vi "Panel.vi"(11 "BooleanIndicatorEditorPanel in":refnum<class "BooleanIndicatorEditorPanel.lvclass">) -> ()   [LabVIEW 2020, in "VolatusGUIControls.lvlib" / "BooleanIndicatorEditorPanel.lvclass"]
uses:
  BooleanIndicatorEditorPanel.lvclass
  BooleanIndicatorEditorPanel.lvclass/BooleanIndicatorEditorPanel.ctl
  lv-oopanel/OOPanel/Panel/Basic UI State.ctl
  lv-oopanel/OOPanel/Panel/Panel.lvclass
  lv-oopanel/OOPanel/OOPanel.lvlib
  VolatusGUIEditorCore/ElementEditorPanel/ElementEditorPanel.lvclass
  lv-autocomplete/AutoComplete/AutoComplete/AutoComplete.lvclass
  VolatusGUIEditorCore/VolatusGUIEditorCore.lvlib
  C:/dev/lv20CE/relink/volatus-gui-controls/VolatusGUIEditorCore/ElementEditorPanel/ElementEditorPanel.lvclass
  C:/dev/lv20CE/relink/lv-oopanel/OOPanel/Panel/Panel.lvclass
  C:/dev/lv20CE/relink/volatus-gui-controls/VolatusGUIControls/BooleanIndicatorEditorPanel/BooleanIndicatorEditorPanel.lvclass
panel:
  in  "Text":bool
  in  "Top":i32
  in  "Left":i32
  in  "Height":u16
  in  "Width":u16
  in  "Label Text Color":u32(colorbox) caption="Color"
  in  "Text Color":u32(colorbox) caption="Color"
  in  "Label Visible":bool caption="Visible"
  in  "Label":string
  in  "Multi":bool
  in  "Channel":string
  in  "True Color":u32(colorbox)
  in  "False Color":u32(colorbox)
  in  "True Text":string
  in  "False Text":string
  # "Label"
  # "False"
  # "True"
  # "LED"
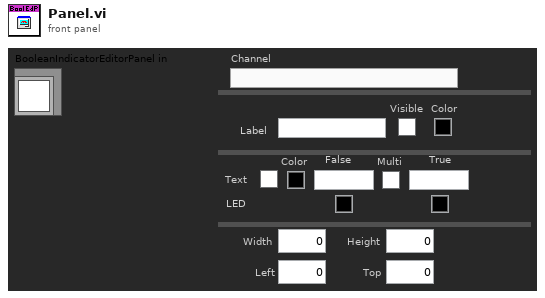
[diagram p1: front panel]
types:
  T1 = typedef "OOPanel.lvlib/Panel.lvclass/Basic UI State.ctl" = enum16{"Init", "Run", "Close"}
  T2 = typedef "VolatusGUIEditorCore.lvlib/ElementEditorPanel.lvclass/Incoming Events.ctl" = cluster{"Update Control":refnum<user-event>}
  T3 = typedef "OOPanel.lvlib/Panel.lvclass/Panel Events.ctl" = cluster{"Visbility":refnum<user-event>, "Close":refnum<user-event>}
  T4 = typedef "VolatusGUIControls.lvlib/BooleanIndicatorEditorPanel.lvclass/Props.ctl" = cluster{"JSON":T5, "Label":T6, "Position":T7, "Width":u16, "Height":u16, "Boolean Colors":T8, "Boolean Text Props":T9}
  T5 = typedef "VolatusGUIControls.lvlib/BooleanIndicatorEditorPanel.lvclass/JSON Props.ctl" = cluster{"Channel":string}
  T6 = typedef "VolatusGUIEditorCore.lvlib/Label Props.ctl" = cluster{"Text":string, "Text Color":u32, "Visible":bool}
  T7 = typedef "VolatusGUIEditorCore.lvlib/Position Props.ctl" = cluster{"Left":i32, "Top":i32}
  T8 = typedef "VolatusGUIEditorCore.lvlib/Boolean Color Props.ctl" = cluster{"False":u32, "True":u32}
  T9 = typedef "VolatusGUIEditorCore.lvlib/Boolean Text Props.ctl" = cluster{"Color":u32, "MultiString":bool, "False":string, "True":string, "Visible":bool}
  T10 = typedef "OOPanel.lvlib/Visibility State.ctl" = enum16{"Idle", "Closed", "Hidden", "Visible", "Subpanel", "Hidden Subpanel"}
  T11 = cluster{"Text Color":u32, "Multi":bool, "False Text":string, "True Text":string, "Text":bool}
  T12 = cluster{"Label":string, "Label Text Color":u32, "Label Visible":bool}
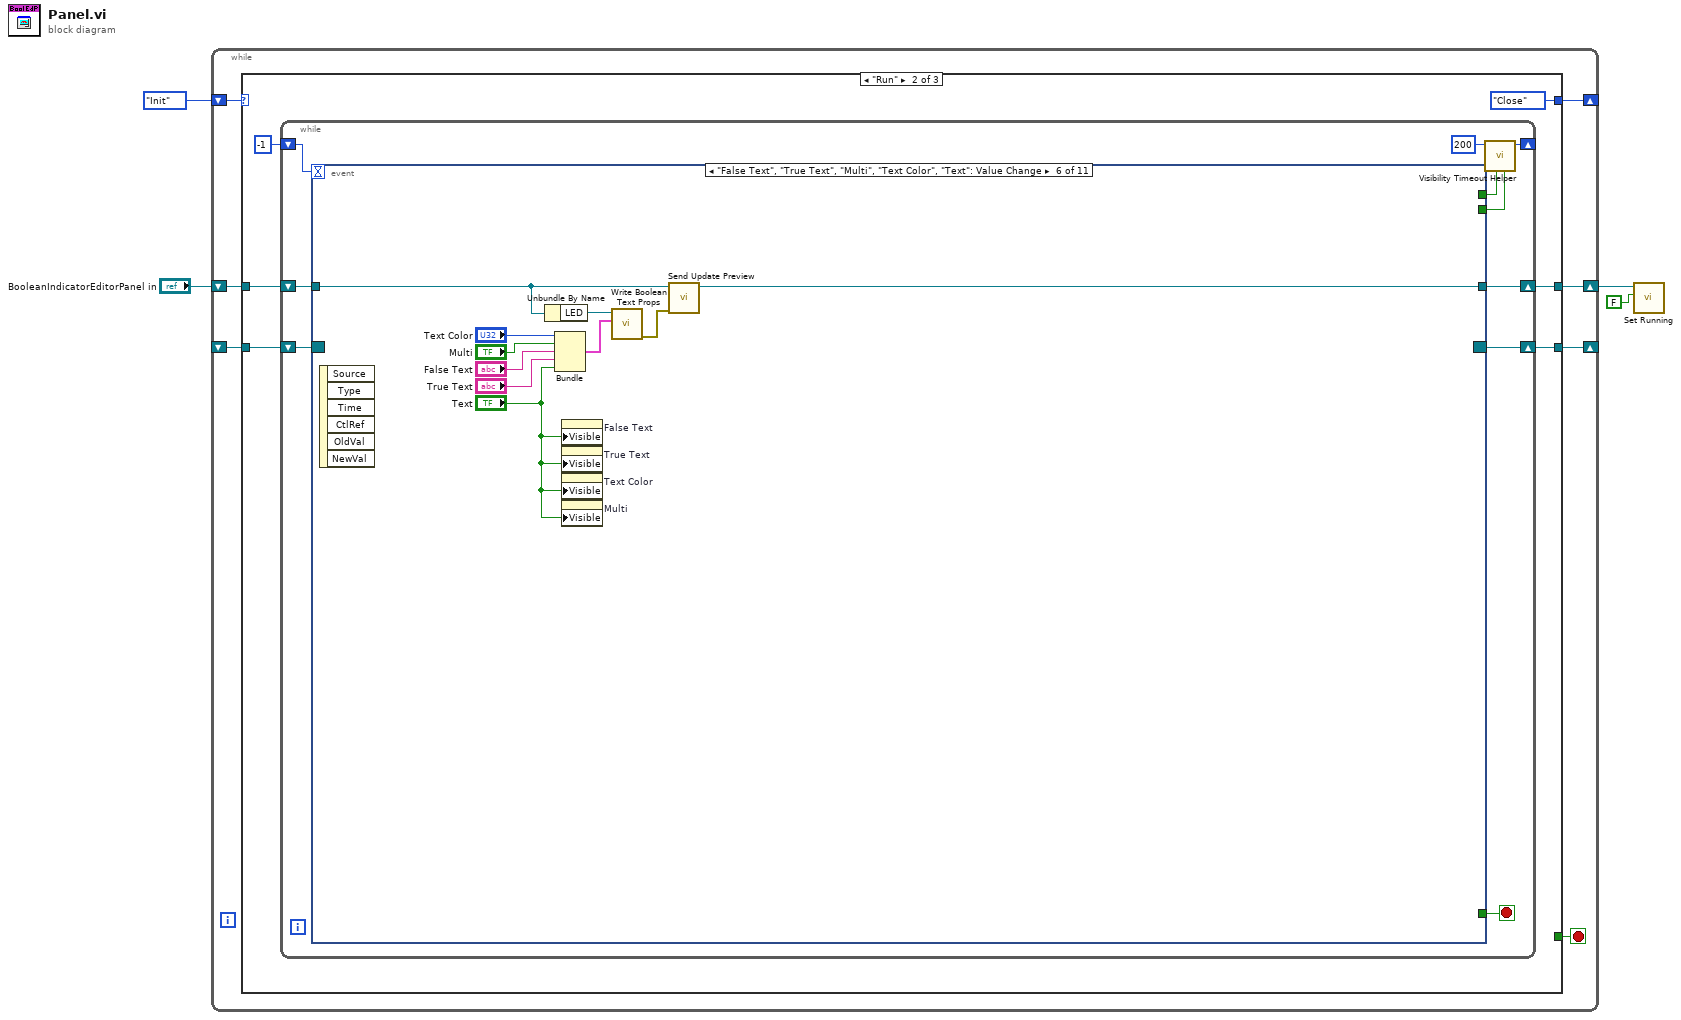
[diagram p0: block diagram]
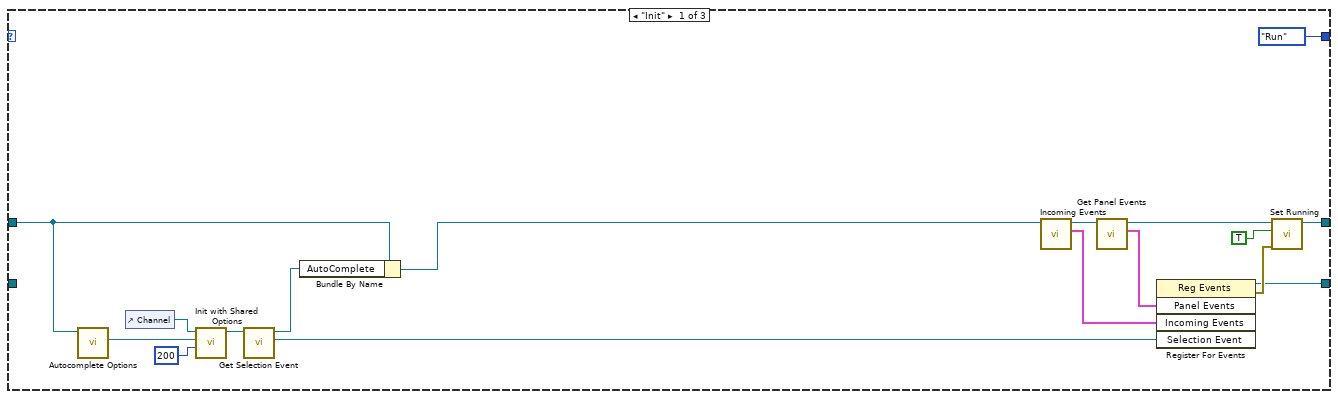
[diagram p2: hidden frame]
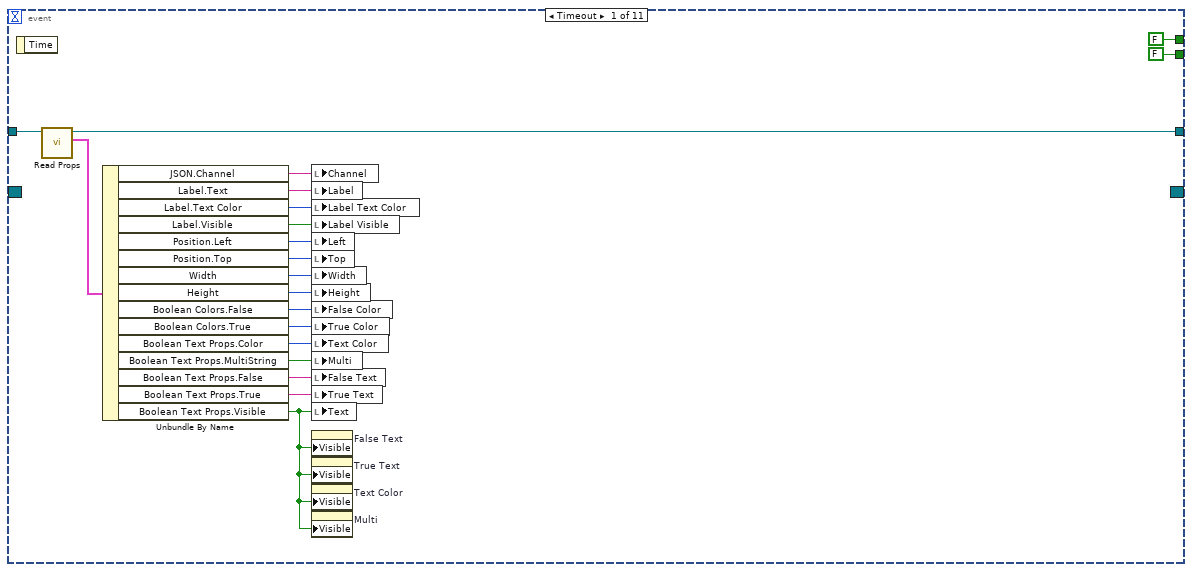
[diagram p3: hidden frame]
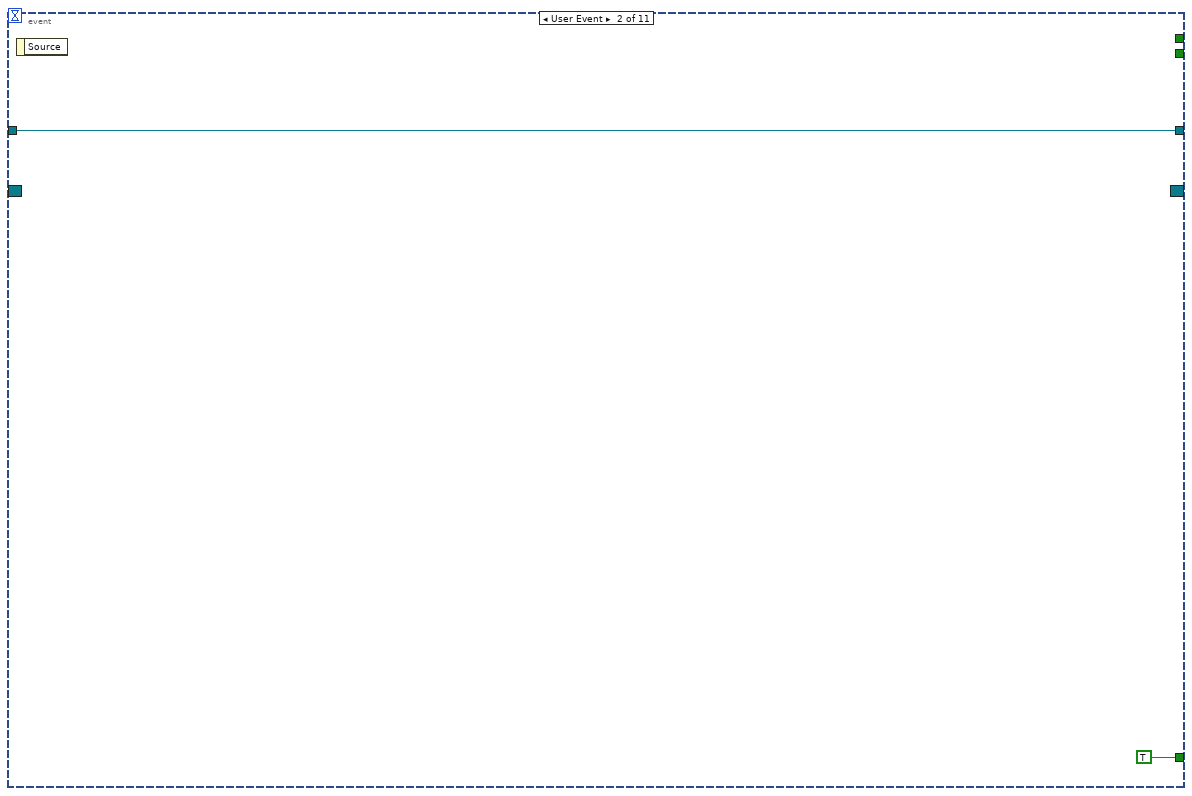
[diagram p4: hidden frame]
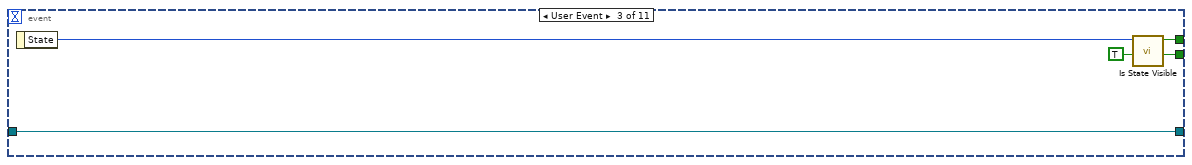
[diagram p5: hidden frame]
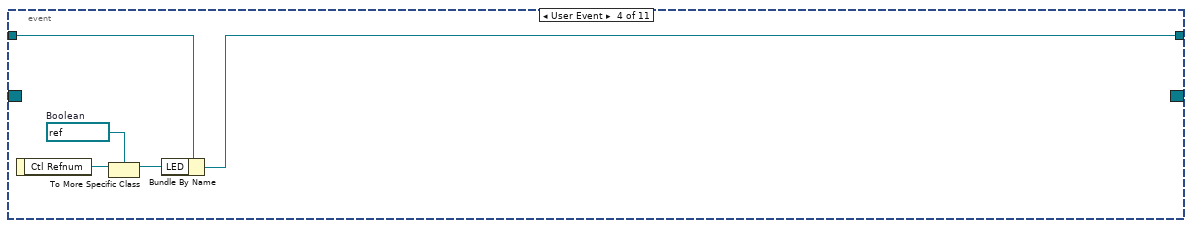
[diagram p6: hidden frame]
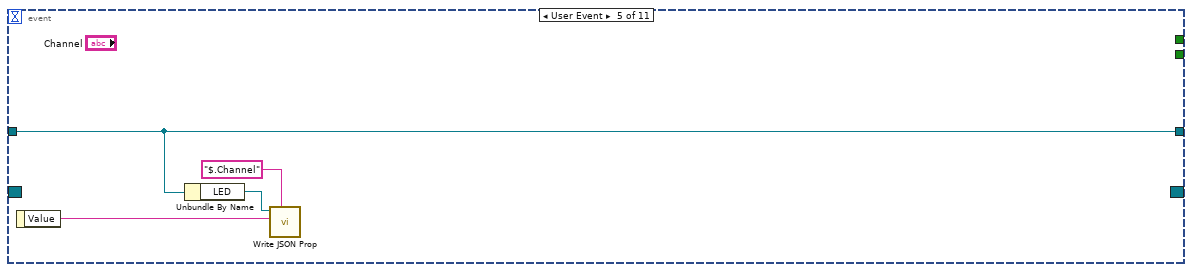
[diagram p7: hidden frame]
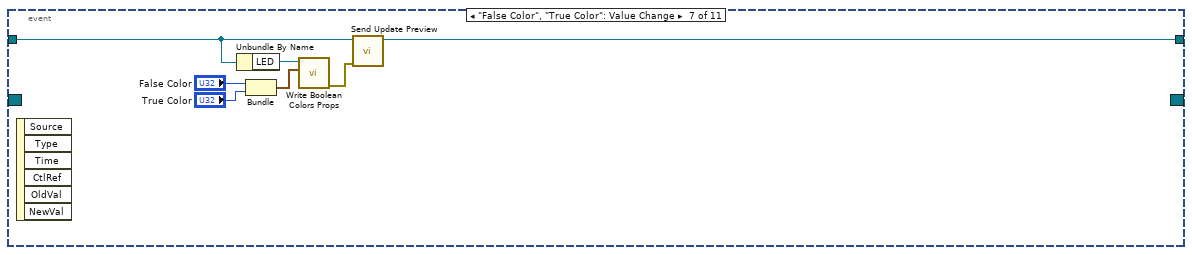
[diagram p8: hidden frame]
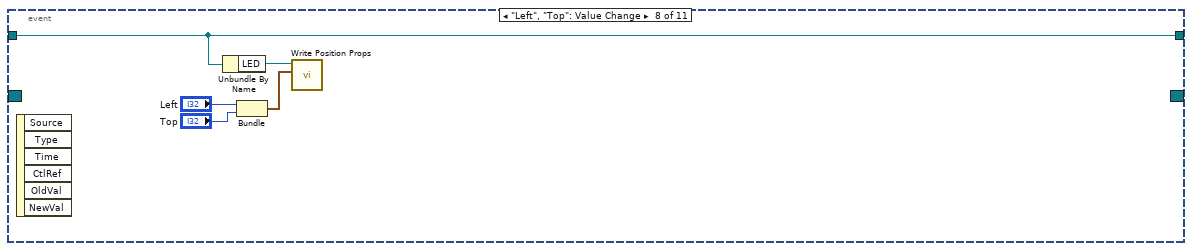
[diagram p9: hidden frame]
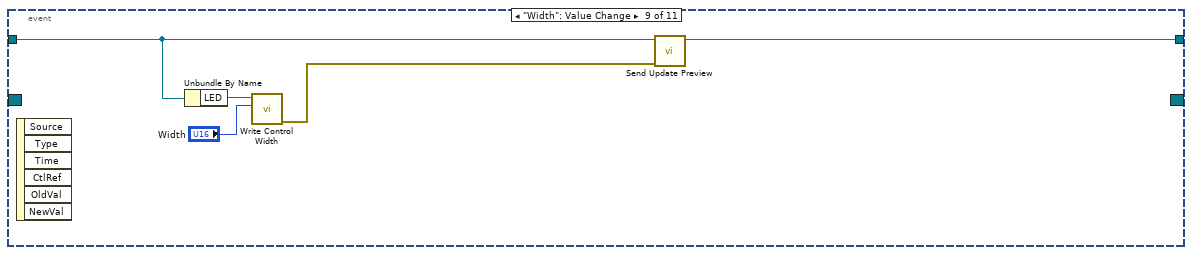
[diagram p10: hidden frame]
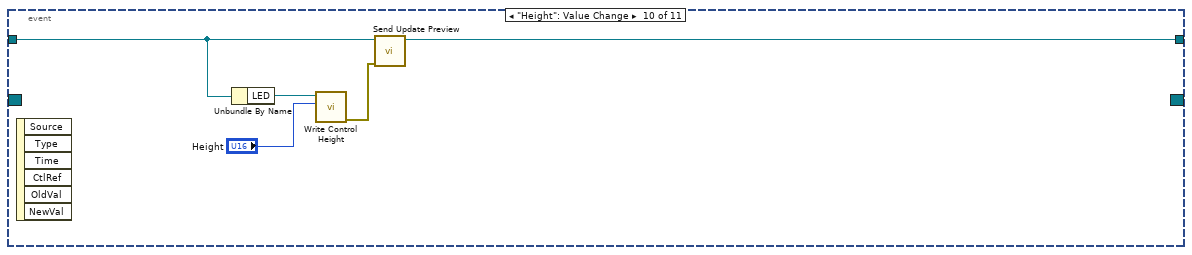
[diagram p11: hidden frame]
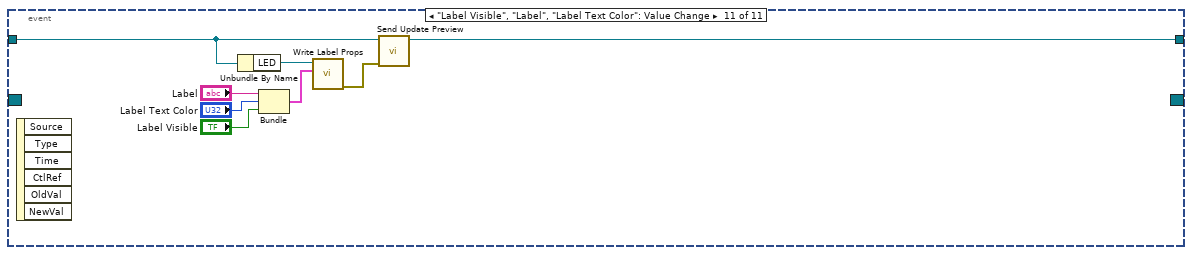
[diagram p12: hidden frame]
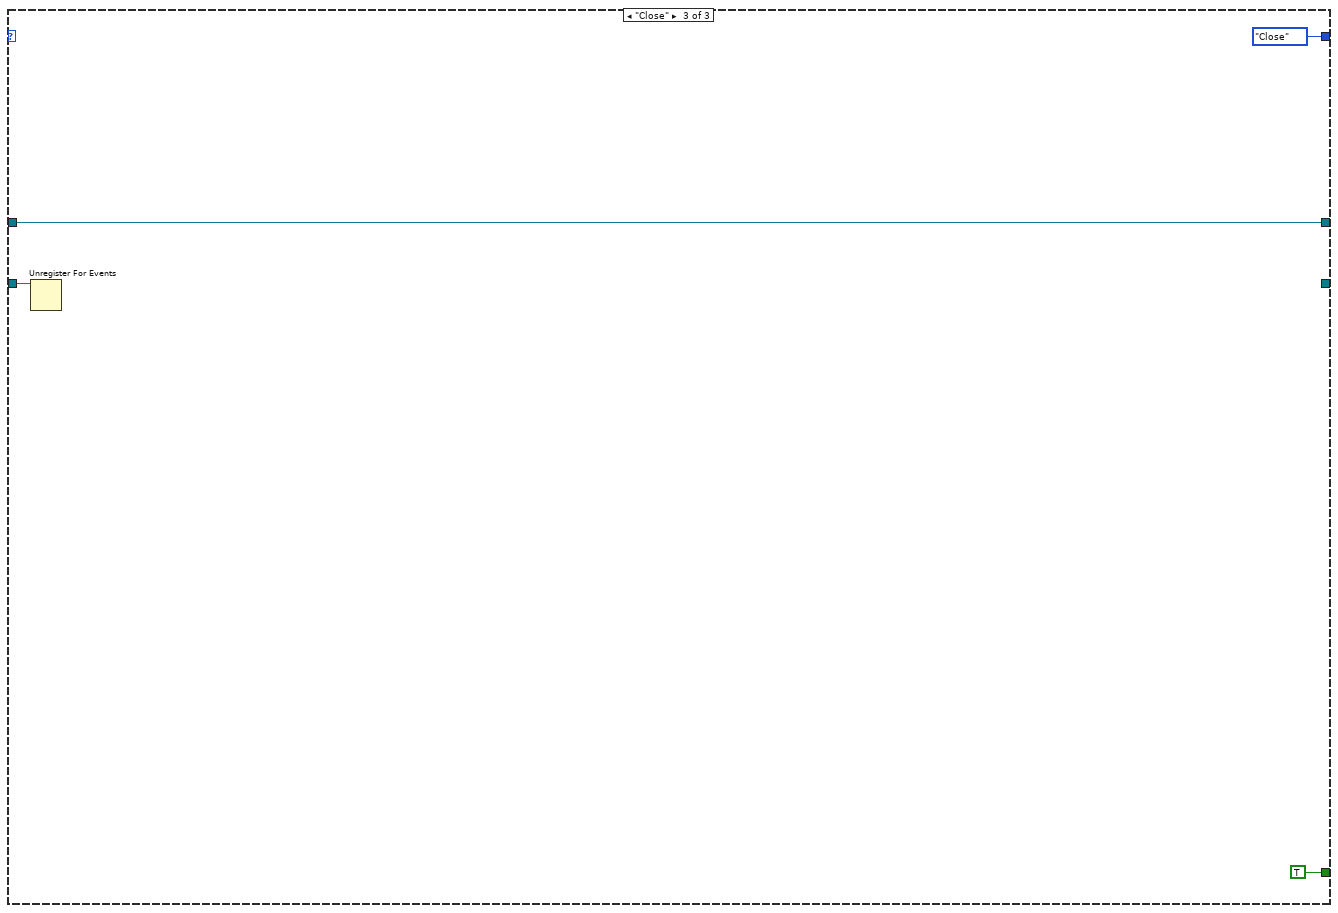
[diagram p13: hidden frame]
diagram:
  n1 = while {
    shift-right: [w10] -> _
    shift-left: _ -> [w11]
    shift-right: [w8] -> _
    shift-left: Basic_UI_State."Init" ("Basic UI State") -> [w9]
    shift-right: [w6] -> w4
    shift-left: "BooleanIndicatorEditorPanel in" -> [w5]
    stop <- w7 stop-if-true
    n2 = case shown="\"Run\"" w9 {
      tunnel: w11 -> [_ w34 w121]
      tunnel: [w25 w32 _] -> w10
      tunnel: [Basic_UI_State."Run" ("Basic UI State") Basic_UI_State."Close" ("Basic UI State") Basic_UI_State."Close" ("Basic UI State")] -> w8
      tunnel: [_ _ TRUE] -> w7
      tunnel: [w24 w29 w120] -> w6
      tunnel: w5 -> [w16 w30 w120]
      frame "Init" {
        n3 = call "Autocomplete Options.vi"("ElementEditorPanel in"=w16) -> ("Autocomplete Options"=w19:refnum<class "Shared Options.lvclass">)  [unwired: 10 in]
        n4 = control-ref of="Channel"() -> (w15:refnum<vi>)
        n5 = call "Init with Shared Options.vi"("Height (200)"=i16 200, "Shared Options"=w19, "Str Refnum"=w15) -> ("AutoComplete out"=w18:refnum<class "AutoComplete.lvclass">)  [unwired: 7 in, 1 out]
        n6 = call "Get Selection Event.vi"("AutoComplete in"=w18) -> ("Selection Event"=w12:refnum<user-event>, "AutoComplete"=w13:refnum<class "AutoComplete.lvclass">)  [unwired: 9 in]
        n7 = Bundle By Name(cluster=w16, "AutoComplete"=w13) -> (w14:refnum<class "BooleanIndicatorEditorPanel.lvclass">)
        n8 = call "Incoming Events.vi"("ElementEditorPanel in"=w14) -> ("Incoming Events"=w20:T2, "ElementEditorPanel out"=w21:refnum<class "BooleanIndicatorEditorPanel.lvclass">)  [unwired: 9 in]
        n9 = call "Get Panel Events.vi"("Panel in"=w21) -> ("Panel Events"=w22:T3, "Panel out"=w23:refnum<class "BooleanIndicatorEditorPanel.lvclass">)  [unwired: 8 in, 1 out]
        n10 = register-events(w22, w20, w12) -> (reference out=w25:refnum<event-registration>, error out=w27:errorcluster)  [unwired: 2 in]
        n11 = call "Set Running.vi"("error in (no error)"=w27, "Running"=TRUE, "Panel in"=w23) -> ("Panel out"=w24:refnum<class "BooleanIndicatorEditorPanel.lvclass">)  [unwired: 7 in, 1 out]
      }
      frame "Run" {
        n12 = while {
          shift-right: [w40] -> w32
          shift-left: w34 -> [w41]
          shift-right: [w43] -> _
          shift-left: -1 ("Timeout") -> [w42]
          shift-right: [w35] -> w29
          shift-left: w30 -> [w36]
          stop <- w37 stop-if-true
          n13 = event shown="[5] \"False Text\", \"True Text\", \"Multi\", \"Text Color\", \"Text\": Value Change" {
            selector: w41 -> [_ _ _ _ _ _ _ _ _ _ _]
            dyn-events: [_ _ _ _ _ _ _ _ _ _ _] -> w40
            timeout: w42 -> [_ _ _ _ _ _ _ _ _ _ _]
            tunnel: [FALSE _ w69 _ _ _ _ _ _ _ _] -> w39
            tunnel: [FALSE _ TRUE _ _ _ _ _ _ _ _] -> w38
            tunnel: [_ TRUE _ _ _ _ _ _ _ _ _] -> w37
            tunnel: w36 -> [w61 w65 w67 w75 w77 w84 w93 w98 w105 w110 w115]
            tunnel: [w62 w65 w67 w72 w77 w82 w91 w98 w103 w108 w113] -> w35
            event Timeout {
              n14 = event-data() -> ()  [unwired: 1 in, 1 out]
              n15 = call "Read Props.vi"("BooleanIndicatorEditorPanel in"=w61) -> ("Props"=w60:T4, "BooleanIndicatorEditorPanel out"=w62:refnum<class "BooleanIndicatorEditorPanel.lvclass">)  [unwired: 8 in, 1 out]
              n16 = Unbundle By Name(w60) -> ("JSON.Channel"=w59:string, "Label.Text"=w58:string, "Label.Text Color"=w57:u32, "Label.Visible"=w56:bool, "Position.Left"=w55:i32, "Position.Top"=w54:i32, "Width"=w53:u16, "Height"=w52:u16, "Boolean Colors.False"=w51:u32, "Boolean Colors.True"=w50:u32, "Boolean Text Props.Color"=w49:u32, "Boolean Text Props.MultiString"=w48:bool, "Boolean Text Props.False"=w47:string, "Boolean Text Props.True"=w46:string, "Boolean Text Props.Visible"=w45:bool)
              n17 = local write "Channel"(w59) -> ()
              n18 = local write "Label"(w58) -> ()
              n19 = local write "Label Text Color"(w57) -> ()
              n20 = local write "Label Visible"(w56) -> ()
              n21 = local write "Left"(w55) -> ()
              n22 = local write "Top"(w54) -> ()
              n23 = local write "Width"(w53) -> ()
              n24 = local write "Height"(w52) -> ()
              n25 = local write "False Color"(w51) -> ()
              n26 = local write "True Color"(w50) -> ()
              n27 = local write "Text Color"(w49) -> ()
              n28 = local write "Multi"(w48) -> ()
              n29 = local write "False Text"(w47) -> ()
              n30 = local write "True Text"(w46) -> ()
              n31 = local write "Text"(w45) -> ()
              n32 = property on="False Text" class="Str"("Visible"=w45) -> ()  [unwired: 2 in, 2 out]
              n33 = property on="True Text" class="Str"("Visible"=w45) -> ()  [unwired: 2 in, 2 out]
              n34 = property on="Text Color" class="ColBox"("Visible"=w45) -> ()  [unwired: 2 in, 2 out]
              n35 = property on="Multi" class="Bool (strict)"("Visible"=w45) -> ()  [unwired: 2 in, 2 out]
            }
            event User Event {
              n36 = event-data() -> ()  [unwired: 1 in, 1 out]
            }
            event User Event {
              n37 = event-data() -> ("State"=w70:T10)  [unwired: 1 in]
              n38 = call "Is State Visible.vi"("Visibility"=w70) -> ("Visible"=w69:bool)  [unwired: 10 in]
            }
            event User Event {
              w73 = refnum<vi> refnum  # Boolean
              n39 = event-data() -> ("Ctl Refnum"=w74:refnum<vi>)  [unwired: 1 in]
              n40 = To More Specific Class(target class=w73, reference=w74) -> (specific class reference=w71:refnum<vi>)  [unwired: 1 in, 1 out]
              n41 = Bundle By Name(cluster=w75, "LED"=w71) -> (w72:refnum<class "BooleanIndicatorEditorPanel.lvclass">)
            }
            event User Event {
              n42 = event-data() -> ("Value"=w76:string)  [unwired: 1 in]
              n43 = Unbundle By Name(w77) -> ("LED"=w79:refnum<vi>)
              n44 = call "Write JSON Prop.vi"("JSON Path"="$.Channel" ("$Path or Item Name"), "Value"=w76, "Ctl Refnum in"=w79) -> ()  [unwired: 7 in, 2 out]
            }
            event "False Text", "True Text", "Multi", "Text Color", "Text": Value Change {
              n45 = event-data() -> ()  [unwired: 1 in, 6 out]
              n46 = Unbundle By Name(w84) -> ("LED"=w83:refnum<vi>)
              n47 = Bundle("Text Color"="Text Color", "Multi"="Multi", "False Text"="False Text", "True Text"="True Text", "Text"="Text") -> (w85:T11)  [unwired: 1 in]
              n48 = property on="False Text" class="Str"("Visible"="Text") -> ()  [unwired: 2 in, 2 out]
              n49 = property on="True Text" class="Str"("Visible"="Text") -> ()  [unwired: 2 in, 2 out]
              n50 = property on="Text Color" class="ColBox"("Visible"="Text") -> ()  [unwired: 2 in, 2 out]
              n51 = property on="Multi" class="Bool (strict)"("Visible"="Text") -> ()  [unwired: 2 in, 2 out]
              n52 = call "Write Boolean Text Props.vi"("Boolean Text Props"=w85, "Control In"=w83) -> ("error out"=w81:errorcluster)  [unwired: 8 in, 1 out]
              n53 = call "Send Update Preview.vi"("error in (no error)"=w81, "ElementEditorPanel in"=w84) -> ("ElementEditorPanel out"=w82:refnum<class "BooleanIndicatorEditorPanel.lvclass">)  [unwired: 8 in, 1 out]
            }
            event "False Color", "True Color": Value Change {
              n54 = event-data() -> ()  [unwired: 1 in, 6 out]
              n55 = Unbundle By Name(w93) -> ("LED"=w92:refnum<vi>)
              n56 = Bundle("False Color"="False Color", "True Color"="True Color") -> (w94:cluster{"False Color":u32, "True Color":u32})  [unwired: 1 in]
              n57 = call "Write Boolean Colors Props.vi"("Boolean Colors Props"=w94, "Control in"=w92) -> ("error out"=w90:errorcluster)  [unwired: 8 in, 1 out]
              n58 = call "Send Update Preview.vi"("error in (no error)"=w90, "ElementEditorPanel in"=w93) -> ("ElementEditorPanel out"=w91:refnum<class "BooleanIndicatorEditorPanel.lvclass">)  [unwired: 8 in, 1 out]
            }
            event "Left", "Top": Value Change {
              n59 = event-data() -> ()  [unwired: 1 in, 6 out]
              n60 = Unbundle By Name(w98) -> ("LED"=w97:refnum<vi>)
              n61 = Bundle("Left"="Left", "Top"="Top") -> (w99:cluster{"Left":i32, "Top":i32})  [unwired: 1 in]
              n62 = call "Write Position Props.vi"("Position Props"=w99, "Ctl Refnum in"=w97) -> ()  [unwired: 8 in, 2 out]
            }
            event "Width": Value Change {
              n63 = event-data() -> ()  [unwired: 1 in, 6 out]
              n64 = Unbundle By Name(w105) -> ("LED"=w104:refnum<vi>)
              n65 = call "Write Control Width.vi"("Width"="Width", "Control in"=w104) -> ("error out"=w102:errorcluster)  [unwired: 8 in, 1 out]
              n66 = call "Send Update Preview.vi"("error in (no error)"=w102, "ElementEditorPanel in"=w105) -> ("ElementEditorPanel out"=w103:refnum<class "BooleanIndicatorEditorPanel.lvclass">)  [unwired: 8 in, 1 out]
            }
            event "Height": Value Change {
              n67 = event-data() -> ()  [unwired: 1 in, 6 out]
              n68 = Unbundle By Name(w110) -> ("LED"=w109:refnum<vi>)
              n69 = call "Write Control Height.vi"("Height"="Height", "Control in"=w109) -> ("error out"=w107:errorcluster)  [unwired: 8 in, 1 out]
              n70 = call "Send Update Preview.vi"("error in (no error)"=w107, "ElementEditorPanel in"=w110) -> ("ElementEditorPanel out"=w108:refnum<class "BooleanIndicatorEditorPanel.lvclass">)  [unwired: 8 in, 1 out]
            }
            event "Label Visible", "Label", "Label Text Color": Value Change {
              n71 = event-data() -> ()  [unwired: 1 in, 6 out]
              n72 = Unbundle By Name(w115) -> ("LED"=w114:refnum<vi>)
              n73 = Bundle("Label"="Label", "Label Text Color"="Label Text Color", "Label Visible"="Label Visible") -> (w116:T12)  [unwired: 1 in]
              n74 = call "Write Label Props.vi"("Label Props"=w116, "Ctl Refnum in"=w114) -> ("error out"=w112:errorcluster)  [unwired: 8 in, 1 out]
              n75 = call "Send Update Preview.vi"("error in (no error)"=w112, "ElementEditorPanel in"=w115) -> ("ElementEditorPanel out"=w113:refnum<class "BooleanIndicatorEditorPanel.lvclass">)  [unwired: 8 in, 1 out]
            }
          }
          n76 = call "Visibility Timeout Helper.vi"("Update?"=w38, "Use Timeout?"=w39, "Visible Timeout mS"=200) -> ("Timeout"=w43:i32)  [unwired: 8 in]
        }
      }
      frame "Close" {
        n77 = Unregister For Events(event registration refnum=w121) -> ()  [unwired: 1 in, 1 out]
      }
    }
  }
  n78 = call "Set Running.vi"("Running"=FALSE, "Panel in"=w4) -> ()  [unwired: 8 in, 2 out]
